vi "Kepco_Test.vi"() -> ()   [LabVIEW 2009]
panel:
  out "Measured Current [A]":dbl
  out "Measured Voltage [V]":dbl
  out "Measured Current [A]":dbl(knob) scale=0.0..10.0
  out "Measured Voltage [V]":dbl(knob) scale=0.0..10.0
  in  "Current [A]":dbl(slide) scale=0.0..2.0
  in  "stop":bool
  in  "RUN":bool
  in  "End Program":bool
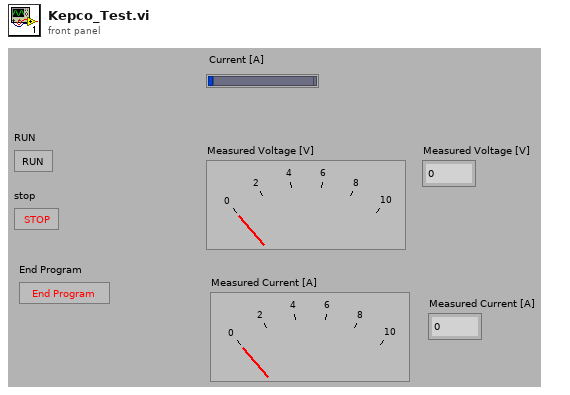
[diagram p1: front panel]
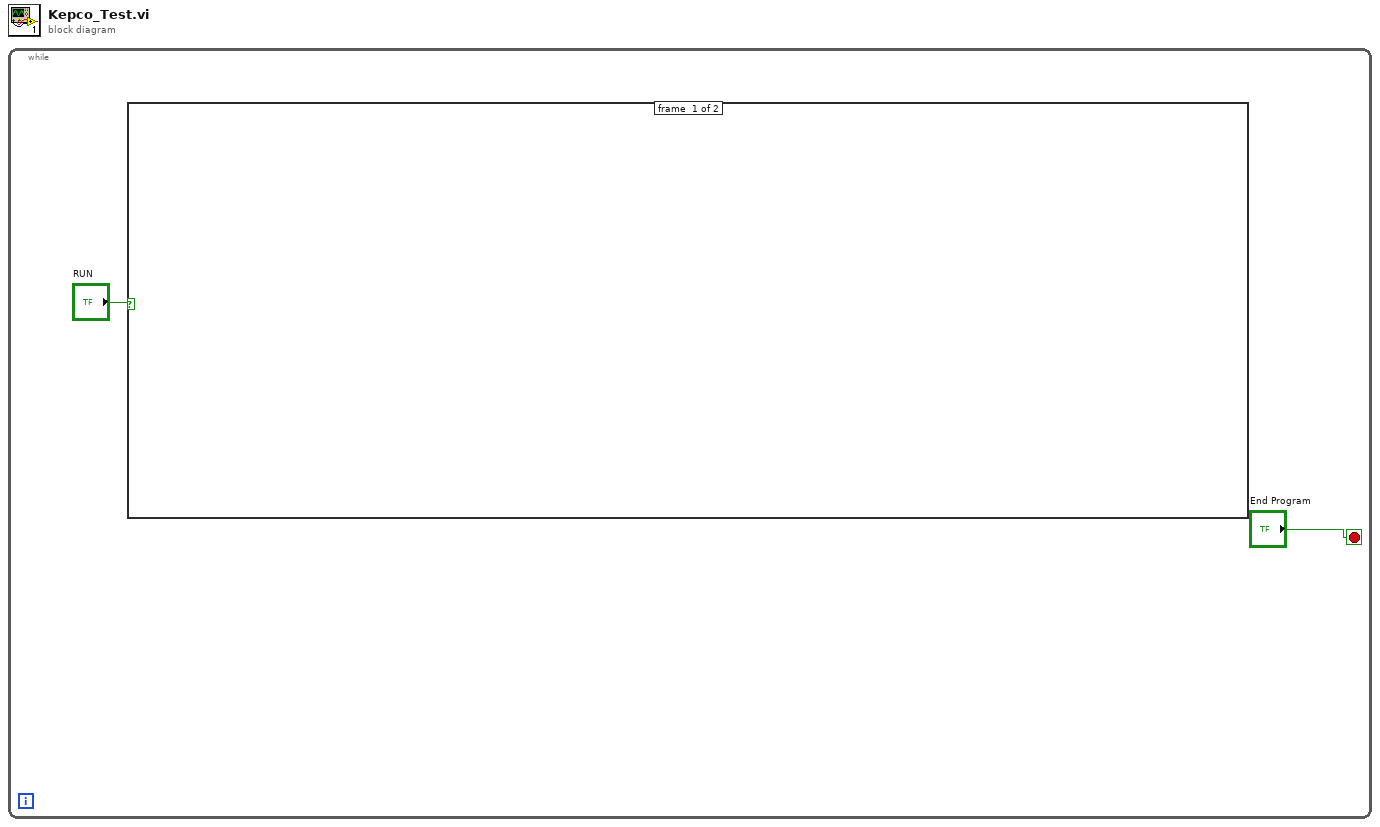
[diagram p0: block diagram]
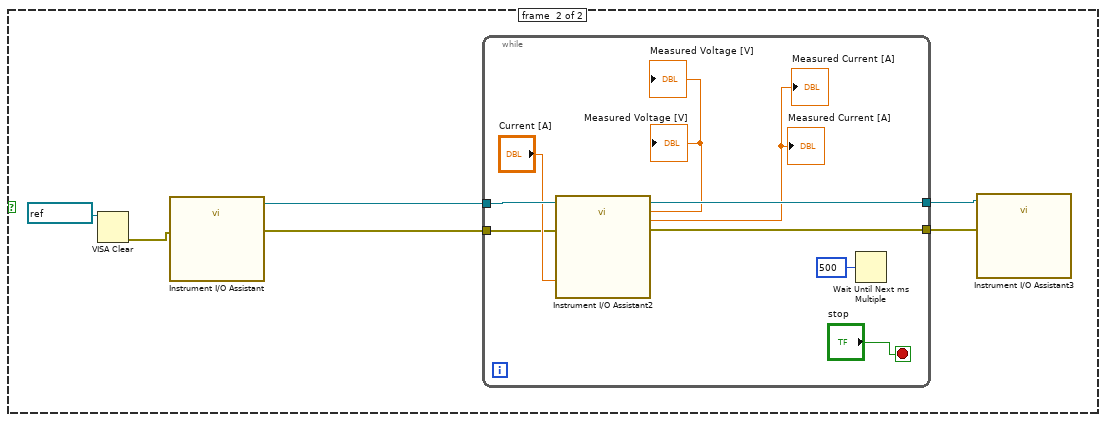
[diagram p2: hidden frame]
diagram:
  n1 = while {
    stop <- "End Program" stop-if-true
    n2 = case shown="True" "RUN" {
      frame #0 {
      }
      frame #1 {
        n3 = VISA Clear(VISA resource name=refnum<visa-resource-name> "COM8") -> (error out=w3:errorcluster)  [unwired: 1 in, 1 out]
        n4 = call "Instrument I/O Assistant"("error in"=w3) -> ("Session Out"=w8:refnum<visa-resource-name>, "error out"=w5:errorcluster)  [unwired: 25 in]
        n5 = while {
          tunnel: w8 -> [w16]
          tunnel: [w14] -> w7
          tunnel: [w13] -> w6
          tunnel: w5 -> [w12]
          stop <- "stop" stop-if-true
          n6 = call "Instrument I/O Assistant2"("Session In"=w16, "Current [A]"="Current [A]", "error in"=w12) -> ("Session Out"=w14:refnum<visa-resource-name>, "Voltage"=→"Measured Voltage [V]" →"Measured Voltage [V]":dbl, "Current"=→"Measured Current [A]" →"Measured Current [A]":dbl, "error out"=w13:errorcluster)  [unwired: 21 in]
          n7 = Wait Until Next ms Multiple(millisecond multiple=u32 500) -> ()  [unwired: 1 out]
        }
        n8 = call "Instrument I/O Assistant3"("Session In"=w7, "error in"=w6) -> ()  [unwired: 24 in, 2 out]
      }
    }
  }
